vi "XYGraphOverview DEMO.vi"() -> ()   [LabVIEW 2020]
uses:
  XYGraphOverview Class/XYGraphOverview.lvclass/XYGraphOverview.ctl
  XYGraphOverview Class/Read X Range Change User Event.vi
  XYGraphOverview Class/Write Block Color.vi
  XYGraphOverview Class/Write Highlight Block Color.vi
  <vilib>/Waveform/WDTOps.llb/WDT Get Waveform Time Array DBL.vi
  XYGraphOverview Class/XYGraphOverview.lvclass
  <vilib>/measure/NI_MABase.lvlib
panel:
  out "All":bool
  out "Upper Range":dbl
  out "Lower Range":dbl
  out "Overview":cluster{"X":dbl[], "Y":dbl[]}[](graph)
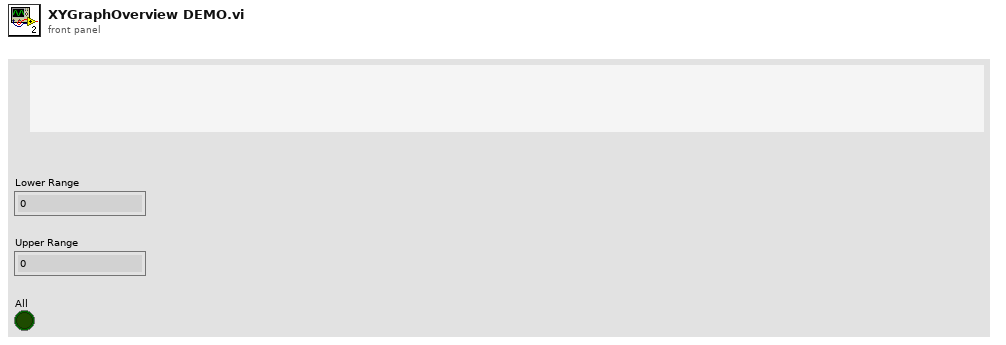
[diagram p1: front panel]
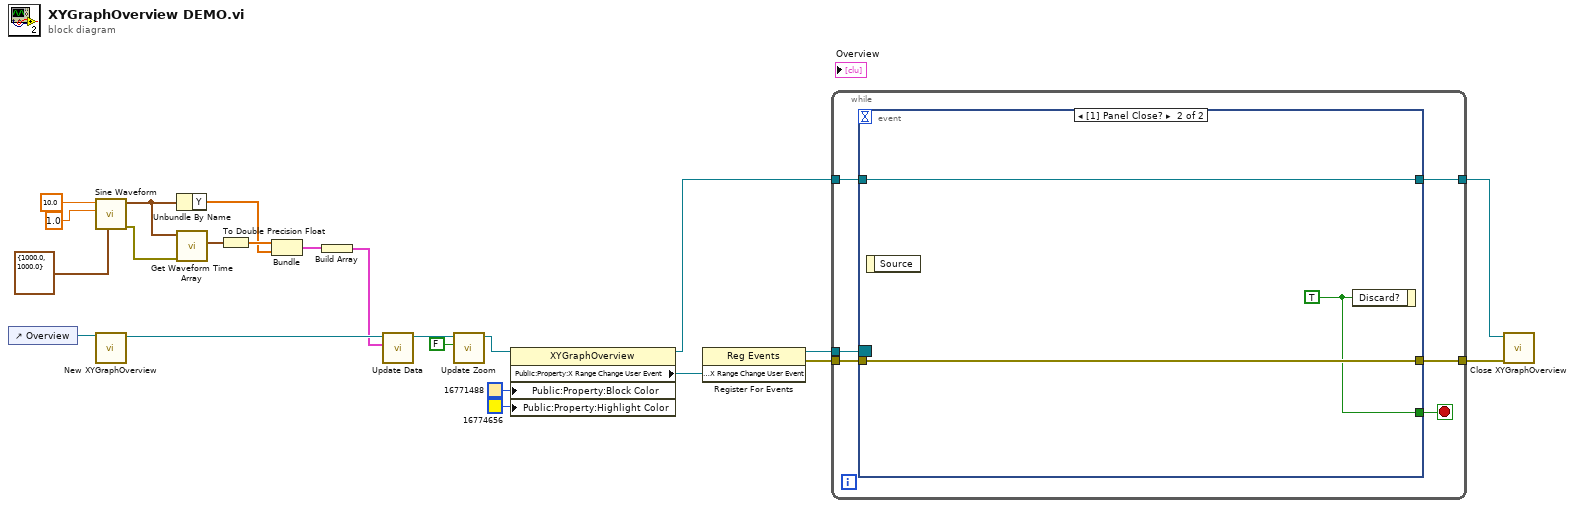
[diagram p0: block diagram]
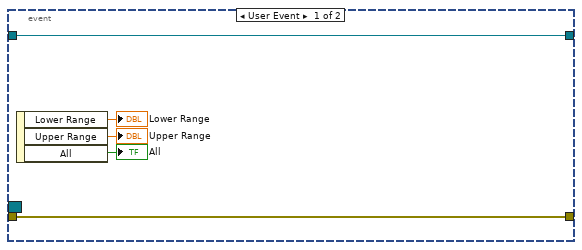
[diagram p2: hidden frame]
diagram:
  n1 = control-ref of="Overview"() -> (w23:refnum<vi>)
  n2 = call <vilib>:"Sine Waveform.vi"("sampling info"=cluster{"Fs":dbl, "#s":dbl} {"Fs"=1000.0, "#s"=1000.0}, "amplitude"=1.0, "frequency"=10.0) -> ("error out"=w18:errorcluster, "signal out"=w17:waveform(dbl))  [unwired: 7 in]
  n3 = call "New XYGraphOverview.vi"("Reference"=w23) -> ("XYGraphOverview out"=w22:refnum<class "XYGraphOverview.lvclass">)  [unwired: 9 in, 1 out]
  n4 = Unbundle By Name(w17) -> ("Y"=w14:dbl[])
  n5 = call-poly <vilib>:"Get Waveform Time Array.vi"("error in (no error)"=w18, "waveform in"=w17) -> ("X array"=w16:timestamp[])  [unwired: 8 in, 1 out]
  n6 = To Double Precision Float(number=w16) -> (double precision float=w15:dbl[])
  n7 = Bundle(w15, "Y"=w14) -> (w13:cluster{dbl[], "Y":dbl[]})  [unwired: 1 in]
  n8 = Build Array(w13) -> (w12:cluster{dbl[], "Y":dbl[]}[])
  n9 = call "Update Data.vi"("Data"=w12, "XYGraphOverview in"=w22) -> ("XYGraphOverview out"=w11:refnum<class "XYGraphOverview.lvclass">)  [unwired: 8 in, 1 out]
  n10 = call "Update Zoom.vi"("Zoom"=FALSE, "XYGraphOverview in"=w11) -> ("XYGraphOverview out"=w9:refnum<class "XYGraphOverview.lvclass">)  [unwired: 8 in, 1 out]
  n11 = property class="XYGraphOverview"(reference=w9, "Public:Property:Block Color"=u32 16771488 ("Block Color"), "Public:Property:Highlight Color"=u32 16774656 ("Highlight Color")) -> (reference out=w5:refnum<class "XYGraphOverview.lvclass">, "Public:Property:X Range Change User Event"=w8:refnum<user-event>)  [unwired: 1 in, 1 out]
  n12 = register-events(w8) -> (reference out=w6:refnum<event-registration>, error out=w7:errorcluster)  [unwired: 2 in]
  n13 = while {
    tunnel: w7 -> [w29]
    tunnel: w6 -> [w28]
    tunnel: w5 -> [w27]
    tunnel: [w26] -> w3
    tunnel: [w25] -> w4
    stop <- w24 stop-if-true
    n14 = event shown="[1] Panel Close?" {
      selector: w28 -> [_ _]
      dyn-events: _ -> [_ _]
      timeout: _ -> [_ _]
      tunnel: w29 -> [w30 w36]
      tunnel: w27 -> [w34 w37]
      tunnel: [w34 w37] -> w26
      tunnel: [w30 w36] -> w25
      tunnel: [_ w35] -> w24
      event User Event {
        n15 = event-data() -> ("Lower Range"=→"Lower Range":dbl, "Upper Range"=→"Upper Range":dbl, "All"=→"All":bool)  [unwired: 1 in]
      }
      event Panel Close? {
        w35 = TRUE ("Discard?")
        n16 = event-data() -> ()  [unwired: 1 in, 1 out]
        n17 = event-data("Discard?"=w35) -> ()  [unwired: 1 in, 1 out]
      }
    }
  }
  n18 = call "Close XYGraphOverview.vi"("error in (no error)"=w4, "XYGraphOverview in"=w3) -> ()  [unwired: 9 in, 1 out]
